vi "IT6322_On_Off.vi"(7 "等待时间(毫秒)":u32=100, 8 "error in":errorcluster caption="错误输入（无错误）", 9 "通道选择":enum16{"第一通道", "第二通道", "第三通道"}(ring), 10 "On_Off":bool, 11 "MyIndex":u8) -> (0 "error out":errorcluster, 3 "状态":bool)   [LabVIEW 2015, in "IT6322.lvlib"]
uses:
  IT6322.lvlib
  <vilib>/Instr/_visa.llb/VISA Configure Serial Port (Instr).vi
panel:
  out "返回值":string
  out "VISA":refnum<visa-resource-name>
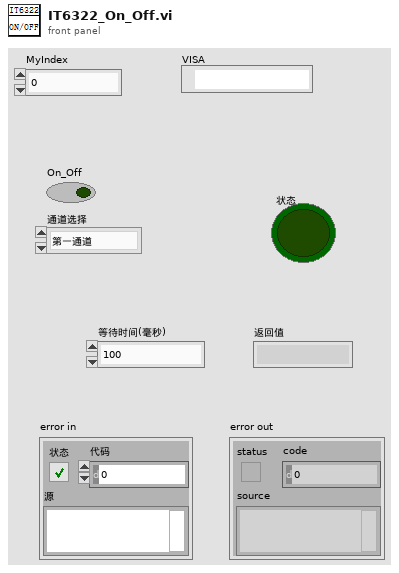
[diagram p1: front panel]
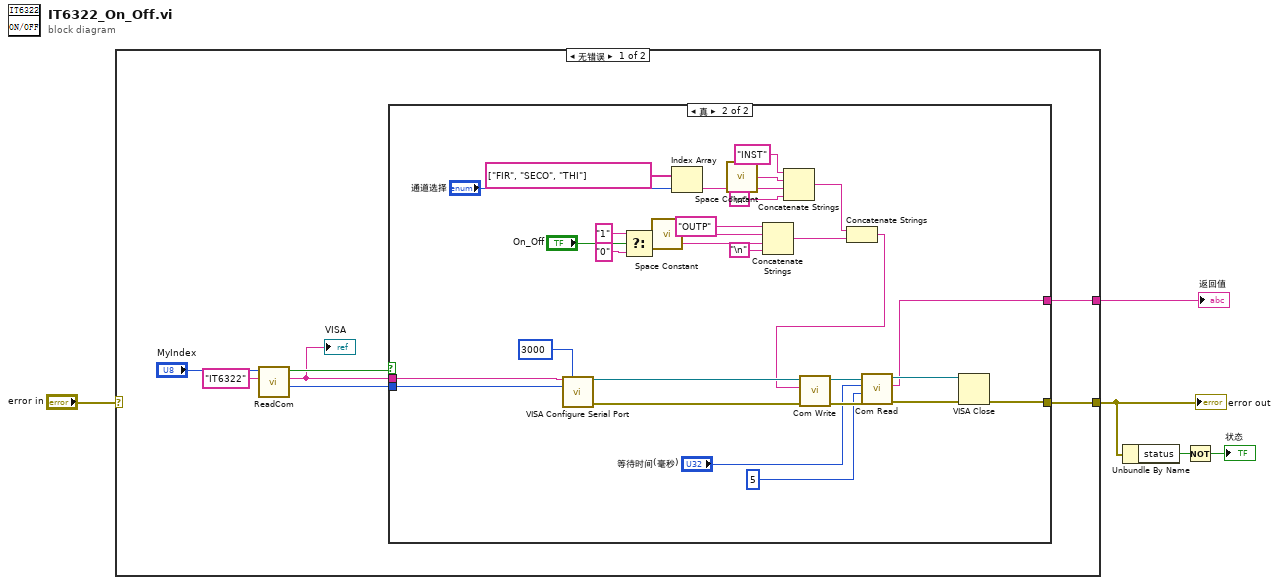
[diagram p0: block diagram]
diagram:
  n1 = case shown="无错误" "error in" {
    selector: "error in" -> [_ w42]
    tunnel: [w12 w42] -> w2
    tunnel: [w6 _] -> w3
    frame No Error {
      n2 = call "ReadCom.vi"("仪器名称"="IT6322", "MyIndex"="MyIndex") -> ("Baudrate"=w7:i32, "COM"=w8:string, "OK?"=w9:bool)  [unwired: 7 in]
      "VISA" <- w8
      n3 = case shown="真" w9 {
        tunnel: [_ w41] -> w12
        tunnel: w8 -> [_ w40]
        tunnel: w7 -> [_ w39]
        tunnel: [_ w31] -> w6
        frame False {
        }
        frame True {
          n4 = call-poly "VISA Configure Serial Port"("VISA resource name"=w40, "timeout (10sec)"=u32 3000, "baud rate (9600)"=w39) -> ("VISA resource name out"=w37:refnum<visa-resource-name>, "error out"=w36:errorcluster)  [unwired: 11 in]
          n5 = Select(t="1", s="On_Off", f="0") -> (s? t:f=w17:string)
          n6 = call <vilib>:"Space Constant.vi"() -> ("String"=w19:string)
          n7 = Index Array(array=string[] ["FIR", "SECO", "THI"], index="通道选择") -> (element=w28:string)
          n8 = call <vilib>:"Space Constant.vi"() -> ("String"=w22:string)
          n9 = Concatenate Strings("OUTP", w19, w17, "\n") -> (w25:string)
          n10 = Concatenate Strings("INST", w22, w28, "\n") -> (w24:string)
          n11 = Concatenate Strings(w24, w25) -> (w13:string)
          n12 = call "Com Write.vi"("错误输入（无错误）"=w36, "Wbuff"=w13, "VISA In"=w37) -> ("错误输出"=w34:errorcluster, "VISA Out"=w35:refnum<visa-resource-name>)  [unwired: 7 in]
          n13 = call "Com Read.vi"("错误输入（无错误）"=w34, "num"=u32 5, "超时"="等待时间(毫秒)", "VISA In"=w35) -> ("错误输出"=w33:errorcluster, "buff"=w31:string, "VISA Out"=w32:refnum<visa-resource-name>)  [unwired: 5 in]
          n14 = VISA Close(VISA resource name=w32, error in (no error)=w33) -> (error out=w41:errorcluster)
        }
      }
    }
    frame Error {
    }
  }
  "error out" <- w2
  "返回值" <- w3
  n15 = Unbundle By Name(w2) -> ("status"=w1:bool)
  n16 = Not(x=w1) -> (.not. x?=→"状态":bool)
